vi "Data Changed.vi"(11 "Data":variant) -> (3 "Changed?":bool)   [LabVIEW 2015]
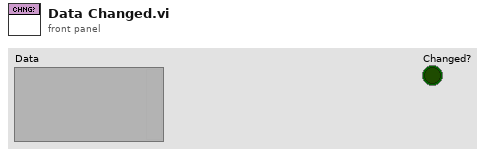
[diagram p1: front panel]
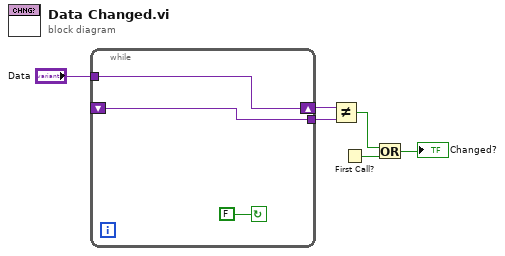
[diagram p0: block diagram]
diagram:
  n1 = while {
    tunnel: "Data" -> [w9]
    shift-right: [w9] -> w5
    shift-left: _ -> [w7]
    tunnel: [w7] -> w4
    stop <- FALSE continue-if-true
  }
  n2 = Not Equal?(x=w5, y=w4) -> (x != y?=w2:bool)
  n3 = First Call?() -> (First Call?: T/F=w3:bool)
  n4 = Or(x=w2, y=w3) -> (x .or. y?=→"Changed?":bool)
